vi "Determination_of_Min_Max_Average_Value.vi"(0 "SI600.lvclass in":refnum<class "SI600.lvclass">, 1 "RCP speed Loop 10":dbl, 2 "RCP speed Loop 20":dbl, 3 "RCP speed Loop 30":dbl, 4 "RCP speed Loop 40":dbl, 5 "error in":errorcluster) -> (14 "SI600.lvclass out":refnum<class "SI600.lvclass">, 15 "RCP Speed Max":dbl, 16 "RCP Speed AVG":dbl, 17 "RCP Speed Min":dbl, 19 "error IO":errorcluster)   [LabVIEW 2022 SP3, in "SI600.lvclass"]
uses:
  SI600.lvclass
  SI600.lvclass/SI600.ctl
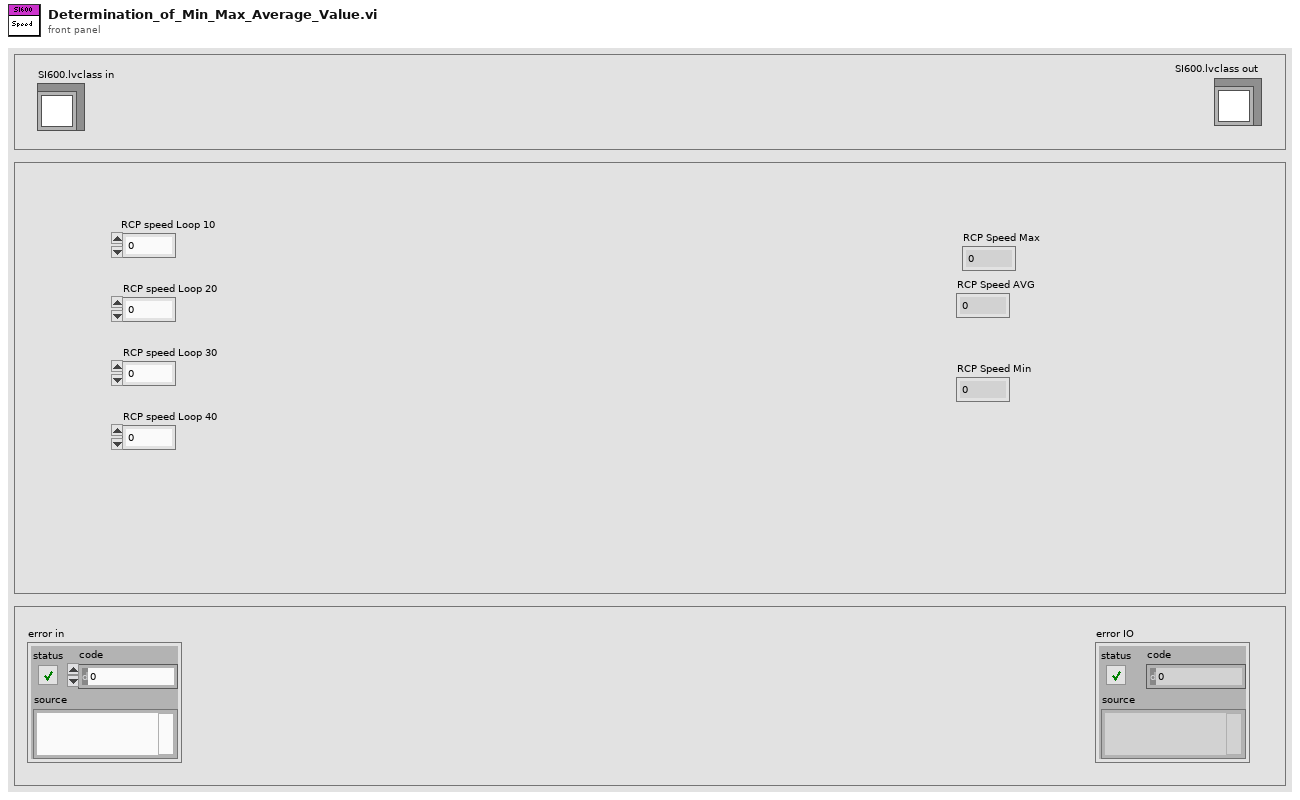
[diagram p1: front panel]
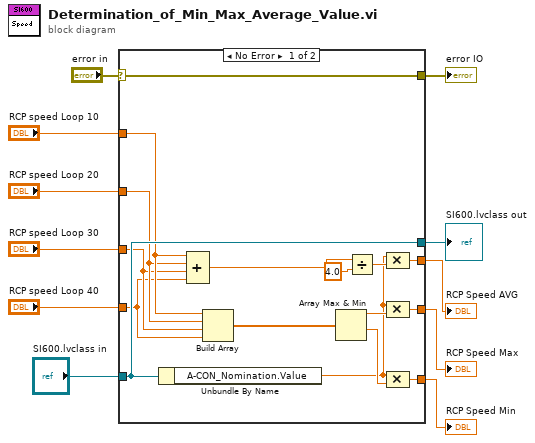
[diagram p0: block diagram]
diagram:
  n1 = case shown="No Error" "error in" {
    selector: "error in" -> [w21 w28]
    tunnel: "SI600.lvclass in" -> [w20 w29]
    tunnel: [w20 w29] -> w9
    tunnel: [w25 _] -> w2
    tunnel: [w24 _] -> w3
    tunnel: [w22 _] -> w1
    tunnel: [w21 w28] -> w8
    tunnel: "RCP speed Loop 10" -> [w18 _]
    tunnel: "RCP speed Loop 20" -> [w17 _]
    tunnel: "RCP speed Loop 30" -> [w16 _]
    tunnel: "RCP speed Loop 40" -> [w15 _]
    frame No Error {
      n2 = Unbundle By Name(w20) -> ("A-CON_Nomination.Value"=w12:dbl)
      n3 = Compound Arithmetic op=ADD(w18, w17, w16, w15) -> (w27:dbl)
      n4 = Build Array(w18, w17, w16, w15) -> (w19:dbl[])
      n5 = Array Max & Min(array=w19) -> (max value=w14:dbl, min value=w13:dbl)  [unwired: 2 out]
      n6 = Divide(x=w27, y=4.0) -> (x/y=w23:dbl)
      n7 = Compound Arithmetic op=MULTIPLY(w12, w23) -> (w22:dbl)
      n8 = Compound Arithmetic op=MULTIPLY(w12, w14) -> (w24:dbl)
      n9 = Compound Arithmetic op=MULTIPLY(w12, w13) -> (w25:dbl)
    }
    frame Error {
    }
  }
  "SI600.lvclass out" <- w9
  "error IO" <- w8
  "RCP Speed Max" <- w3
  "RCP Speed Min" <- w2
  "RCP Speed AVG" <- w1
